vi "set_z.vi"(8 "error in":errorcluster, 11 "z_value_um":dbl format="%0.2f") -> (0 "error out":errorcluster)   [LabVIEW 2018]
uses:
  <vilib>/DAQmx/write.llb/DAQmx Write (Analog DBL 1Chan 1Samp).vi
  GLOBAL_VAR.vi
  <vilib>/DAQmx/create/channels.llb/DAQmx Create Channel (AO-Voltage-Basic).vi
  <vilib>/DAQmx/miscellaneous.llb/DAQmx Fill In Error Info.vi
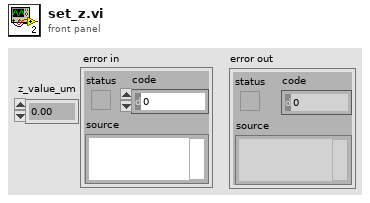
[diagram p1: front panel]
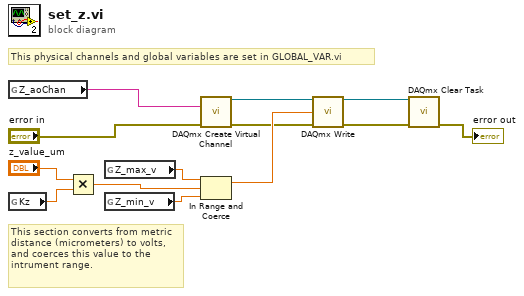
[diagram p0: block diagram]
diagram:
  # "This section converts from metric distance (micrometers) to volts, and coerces this value to the intrument range."
  # "This physical channels and global variables are set in GLOBAL_VAR.vi"
  n1 = global read "GLOBAL_VAR.vi" "Z_aoChan"() -> (w12:tag)
  n2 = global read "GLOBAL_VAR.vi" "Kz"() -> (w9:dbl)
  n3 = Multiply(x="z_value_um", y=w9) -> (x*y=w5:dbl)
  n4 = global read "GLOBAL_VAR.vi" "Z_max_v"() -> (w7:dbl)
  n5 = global read "GLOBAL_VAR.vi" "Z_min_v"() -> (w6:dbl)
  n6 = call-poly <vilib>:"DAQmx Create Virtual Channel.vi"("physical channels"=w12, "error in"="error in") -> ("task out"=w10:refnum<k21>, "error out"=w3:errorcluster)  [unwired: 12 in]
  n7 = In Range and Coerce(upper limit=w7, x=w5, lower limit=w6) -> (coerced(x)=w13:dbl)  [unwired: 1 out]
  n8 = call-poly <vilib>:"DAQmx Write.vi"("task/channels in"=w10, "data"=w13, "error in"=w3) -> ("task out"=w11:refnum<k21>, "error out"=w2:errorcluster)  [unwired: 10 in, 1 out]
  n9 = call <vilib>:"DAQmx Clear Task.vi"("task in"=w11, "error in"=w2) -> ("error out"=→"error out":errorcluster)  [unwired: 13 in]
